vi "Deal_Data2nd.vi"(0 "mbfDealData":bool=TRUE, 1 "ArrayIn":u8[](array[numeric])=[90, 165, 142, 1, 240, 0, 1, 99, 48, 2, 0, 221, 3, 0, 233, 7, 0, 253, 11, 0, 0, 12, 0, 0, 13, 0, 0, 14, 0, 0, 21, 0, 0, 22, 0, 0, 23, 0, 0, 24, 146, 242, 29, 0, 0, 0, 0, 31, 0, 0, 33, 0, 34, 1, 64, 35, 0, 41, 0, 42, 0, 43, 0, 44, 46, 204, 45, 0, 0, 46, 0, 240, 47, 240, 48, 0, 49, 0, 50, 128, 51, 0, 52, 0, 53, 0, 54, 68, 58, 0, 59, 0, 60, 241, 61, 32, 32, 32, 32, 82, 64, 73, 83, 0, 0, 4, 0, 3, 6, 0, 0, 0, 0, 18, 0, 0, 0, 0, 201, 113, 49, 49, 52, 202, 70, 52, 48, 53, 203, 57, 48, 48, 66, 204, 32, 32, 48, 53, 251, 6, 25, 90]) -> (2 "BufSize":u8, 3 "ReferenceArray":string[][](array[string]), 4 "strArrayYesOrNo":string[](array[string]), 5 "strData":string[](array[string]), 6 "BufSize2":u8)   [LabVIEW 2011]
panel:
  in  "mu16CountI":u16
  in  "mu16Count":u16
  out "子数组":string[](array[string])
  out "数组":string[][](array[string])
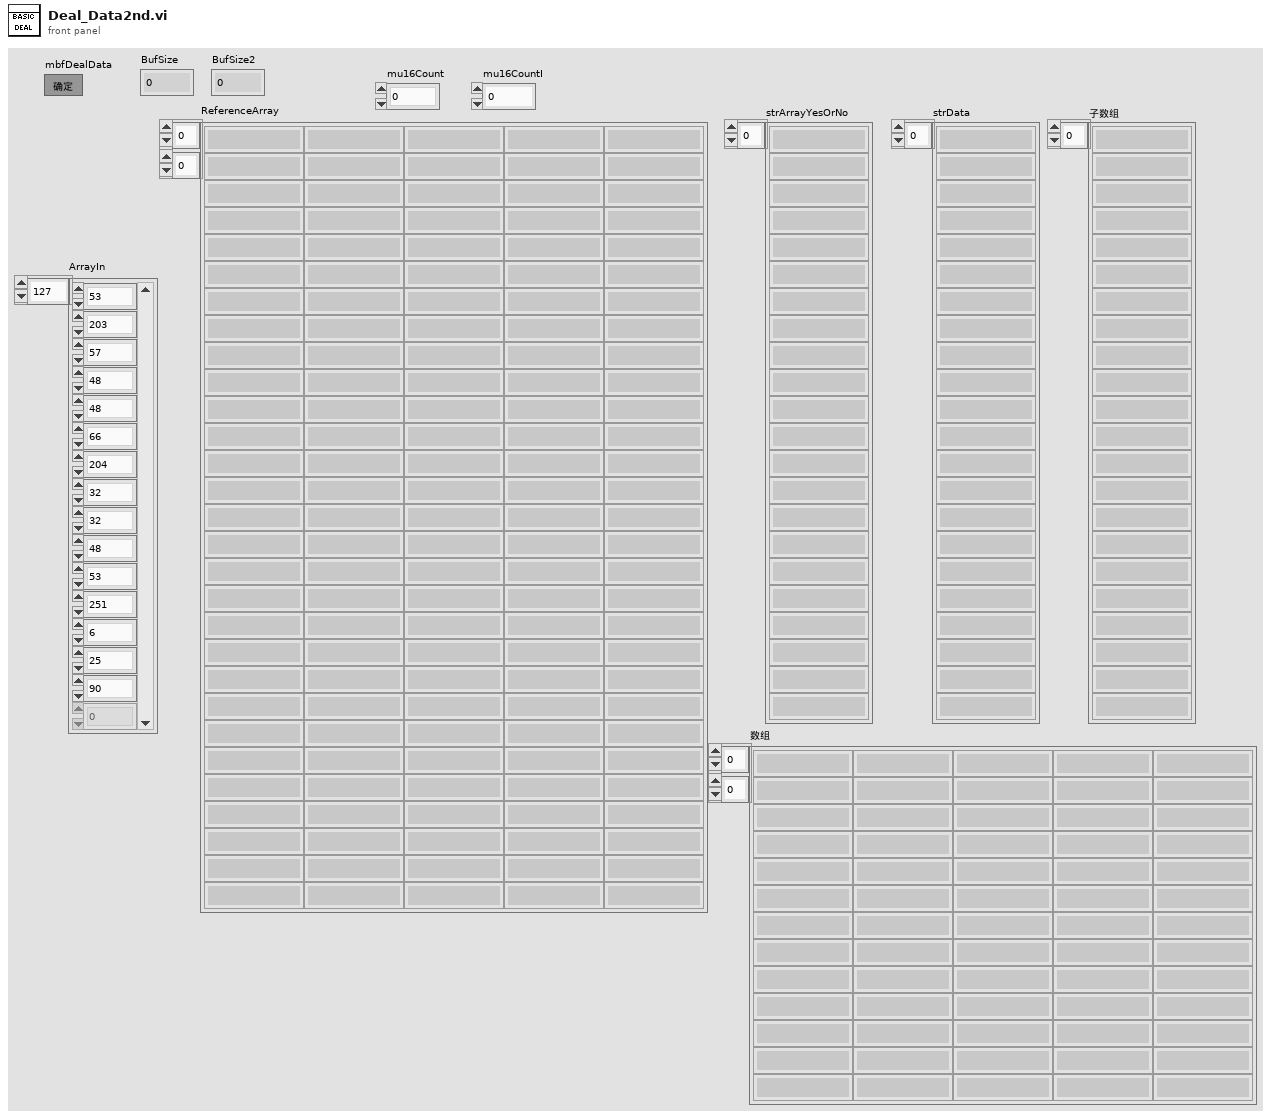
[diagram p1: front panel]
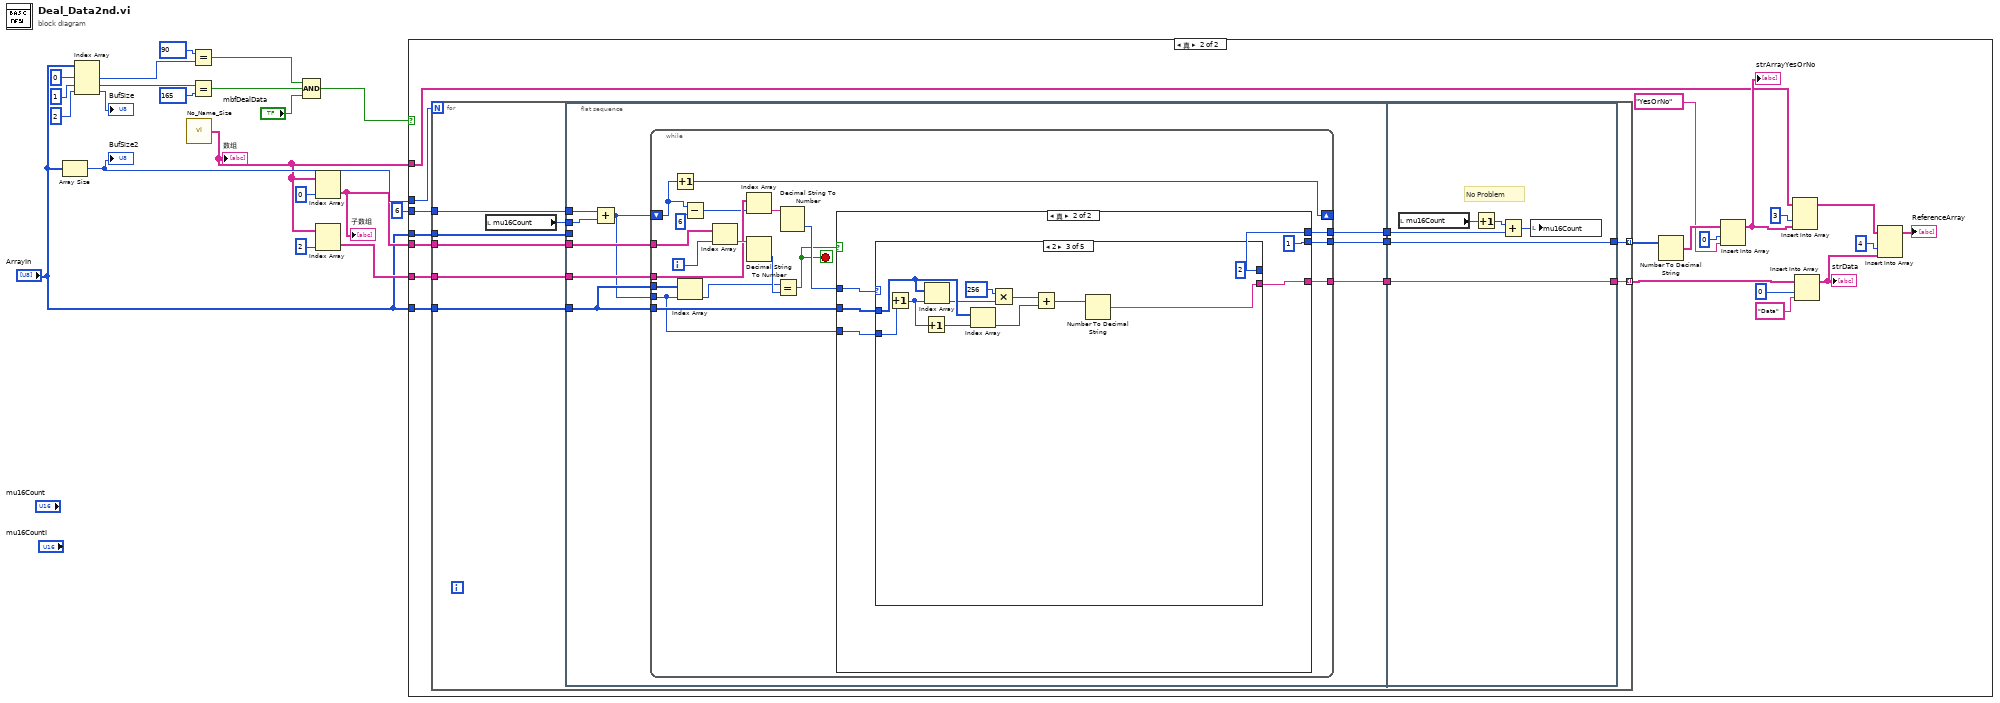
[diagram p0: block diagram]
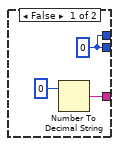
[diagram p3: hidden frame]
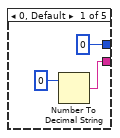
[diagram p4: hidden frame]
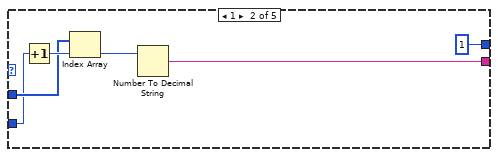
[diagram p5: hidden frame]
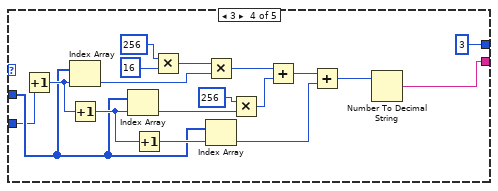
[diagram p6: hidden frame]
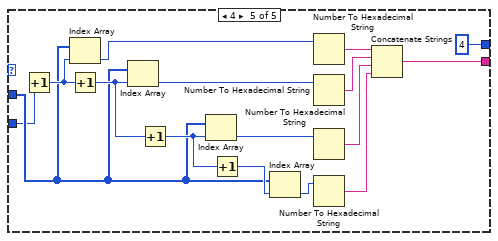
[diagram p7: hidden frame]
diagram:
  n1 = Array Size(array="ArrayIn") -> (size(s)=w5:i32)
  "BufSize2" <- w5
  n2 = Index Array(array="ArrayIn", index #1=0 ("索引"), index #2=1 ("索引"), index #3=2 ("索引")) -> (element #1=w15:u8, element #2=w14:u8, element #3=→"BufSize":u8)
  n3 = call "No_Name_Size.vi"() -> ("数组"=w1:string[][])
  "数组" <- w1
  n4 = Equal?(x=u8 90, y=w15) -> (x = y?=w13:bool)
  n5 = Equal?(x=w14, y=u8 165) -> (x = y?=w12:bool)
  n6 = Compound Arithmetic op=AND(w13, w12, "mbfDealData") -> (w10:bool)
  n7 = Index Array(array=w1, index (col)=0 ("禁用的索引 (列)")) -> (element=w4:string[])  [unwired: 1 in]
  "子数组" <- w4
  n8 = Index Array(array=w1, index (col)=2 ("禁用的索引 (列)")) -> (element=w3:string[])  [unwired: 1 in]
  n9 = case shown="真" w10 {
    tunnel: w5 -> [_ w40]
    tunnel: 6 -> [_ w31]
    tunnel: w4 -> [_ w30]
    tunnel: "ArrayIn" -> [_ w29]
    tunnel: w3 -> [_ w28]
    tunnel: "ArrayIn" -> [_ w26]
    tunnel: w1 -> [_ w24]
    frame False {
    }
    frame True {
      n10 = for {
        N: w40 -> [_]
        tunnel: w31 -> [w51]
        tunnel: w30 -> [w49]
        tunnel: w29 -> [w48]
        tunnel: w28 -> [w47]
        tunnel: [w44] -> w27 mode=indexing
        tunnel: w26 -> [w43]
        tunnel: [w42] -> w25 mode=indexing
        n11 = local read "mu16Count"() -> (w50:u16)
        n12 = flat-sequence {
          tunnel: w51 -> [w60]
          tunnel: w50 -> [w53]
          tunnel: w49 -> [w59]
          tunnel: w48 -> [_]
          tunnel: w47 -> [w58]
          tunnel: [w57] -> w46
          tunnel: [w56] -> w45
          tunnel: w43 -> [w54]
          tunnel: [w55] -> w41
          tunnel: w46 -> [w146]
          tunnel: w45 -> [w144]
          tunnel: [w144] -> w44
          tunnel: [w143] -> w42
          tunnel: w41 -> [w143]
          frame #0 {
            n13 = Add(x=w60, y=w53) -> (x+y=w52:i32)
            n14 = while {
              tunnel: w59 -> [w79]
              tunnel: w58 -> [w76]
              tunnel: [w73] -> w57
              tunnel: [w72] -> w56
              tunnel: w54 -> [w71]
              shift-right: [w70] -> _
              shift-left: w52 -> [w65]
              tunnel: [w69] -> w55
              tunnel: w54 -> [w63]
              tunnel: w52 -> [w61]
              i -> [w62]
              stop <- w68 stop-if-true
              n15 = Increment(x=w65) -> (x+1=w70:i32)
              n16 = Index Array(array=w63, index=w61) -> (element=w64:u8)
              n17 = Subtract(x=w65, y=6) -> (x-y=w66:i32)
              n18 = Index Array(array=w79, index=w62) -> (element=w78:string)
              n19 = Index Array(array=w76, index=w66) -> (element=w75:string)
              n20 = Decimal String To Number(string=w78) -> (number=w77:i32)  [unwired: 2 in, 1 out]
              n21 = Equal?(x=w64, y=w77) -> (x = y?=w68:bool)
              n22 = Decimal String To Number(string=w75) -> (number=w74:i32)  [unwired: 2 in, 1 out]
              n23 = case shown="真" w68 {
                tunnel: [w80 1] -> w72
                tunnel: [w81 w87] -> w69
                tunnel: [w80 w86] -> w73
                tunnel: w74 -> [_ w85]
                tunnel: w71 -> [_ w84]
                tunnel: w61 -> [_ w83]
                frame False {
                  w80 = 0
                  n24 = Number To Decimal String(number=0) -> (decimal integer string=w81:string)  [unwired: 1 in]
                }
                frame True {
                  n25 = case shown="2" w85 {
                    tunnel: [w90 w96 w103 w115 w134] -> w87
                    tunnel: [0 1 2 3 4] -> w86
                    tunnel: w84 -> [_ w94 w101 w113 w132]
                    tunnel: w83 -> [_ w92 w98 w109 w127]
                    frame 0, Default {
                      n26 = Number To Decimal String(number=0) -> (decimal integer string=w90:string)  [unwired: 1 in]
                    }
                    frame 1 {
                      n27 = Increment(x=w92) -> (x+1=w97:i32)
                      n28 = Index Array(array=w94, index=w97) -> (element=w93:u8)
                      n29 = Number To Decimal String(number=w93) -> (decimal integer string=w96:string)  [unwired: 1 in]
                    }
                    frame 2 {
                      n30 = Increment(x=w98) -> (x+1=w107:i32)
                      n31 = Increment(x=w107) -> (x+1=w108:i32)
                      n32 = Index Array(array=w101, index=w107) -> (element=w100:u8)
                      n33 = Index Array(array=w101, index=w108) -> (element=w99:u8)
                      n34 = Multiply(x=u16 256, y=w100) -> (x*y=w105:u16)
                      n35 = Add(x=w105, y=w99) -> (x+y=w104:u16)
                      n36 = Number To Decimal String(number=w104) -> (decimal integer string=w103:string)  [unwired: 1 in]
                    }
                    frame 3 {
                      n37 = Increment(x=w109) -> (x+1=w126:i32)
                      n38 = Index Array(array=w113, index=w126) -> (element=w112:u8)
                      n39 = Increment(x=w126) -> (x+1=w119:i32)
                      n40 = Index Array(array=w113, index=w119) -> (element=w111:u8)
                      n41 = Increment(x=w119) -> (x+1=w118:i32)
                      n42 = Multiply(x=u16 256, y=u16 16 ("x")) -> (x*y=w123:u16)
                      n43 = Multiply(x=w123, y=w112) -> (x*y=w121:u16)
                      n44 = Index Array(array=w113, index=w118) -> (element=w110:u8)
                      n45 = Multiply(x=u16 256, y=w111) -> (x*y=w120:u16)
                      n46 = Add(x=w121, y=w120) -> (x+y=w117:u16)
                      n47 = Add(x=w117, y=w110) -> (x+y=w116:u16)
                      n48 = Number To Decimal String(number=w116) -> (decimal integer string=w115:string)  [unwired: 1 in]
                    }
                    frame 4 {
                      n49 = Increment(x=w127) -> (x+1=w142:i32)
                      n50 = Index Array(array=w132, index=w142) -> (element=w131:u8)
                      n51 = Increment(x=w142) -> (x+1=w141:i32)
                      n52 = Index Array(array=w132, index=w141) -> (element=w130:u8)
                      n53 = Increment(x=w141) -> (x+1=w140:i32)
                      n54 = Index Array(array=w132, index=w140) -> (element=w129:u8)
                      n55 = Increment(x=w140) -> (x+1=w139:i32)
                      n56 = Index Array(array=w132, index=w139) -> (element=w128:u8)
                      n57 = Number To Hexadecimal String(2:w131) -> (0:w138:string)  [unwired: 1 in]
                      n58 = Number To Hexadecimal String(2:w130) -> (0:w137:string)  [unwired: 1 in]
                      n59 = Number To Hexadecimal String(2:w129) -> (0:w136:string)  [unwired: 1 in]
                      n60 = Number To Hexadecimal String(2:w128) -> (0:w135:string)  [unwired: 1 in]
                      n61 = Concatenate Strings(w138, w137, w136, w135) -> (w134:string)
                    }
                  }
                }
              }
            }
          }
          frame #1 {
            # "No Problem"
            n62 = local read "mu16Count"() -> (w148:u16)
            n63 = Increment(x=w148) -> (x+1=w147:u16)
            n64 = Add(x=w147, y=w146) -> (x+y=w145:i32)
            n65 = local write "mu16Count"(w145) -> ()
          }
        }
      }
      n66 = Number To Decimal String(number=w27) -> (decimal integer string=w39:string[])  [unwired: 1 in]
      n67 = Insert Into Array(array=w39, index=0 ("索引"), new element="YesOrNo" ("新元素/子数组")) -> (w36:string[])
      "strArrayYesOrNo" <- w36
      n68 = Insert Into Array(array=w24, index (col)=3 ("索引"), new element=w36) -> (w34:string[][])  [unwired: 1 in]
      n69 = Insert Into Array(array=w25, index=0 ("索引"), new element="Data" ("新元素/子数组")) -> (w22:string[])
      "strData" <- w22
      n70 = Insert Into Array(array=w34, index (col)=4 ("禁用的索引 (列)"), new element=w22) -> (→"ReferenceArray":string[][])  [unwired: 1 in]
    }
  }
